vi "Update.vi"(9 "log line":string, 10 "file ref":refnum<file>, 11 "size trigger in":refnum<class "RolloverTrigger.Size.lvclass">) -> (3 "size trigger out":refnum<class "RolloverTrigger.Size.lvclass">)   [LabVIEW 2018, in "GLog.lvlib" / "RolloverTrigger.Size.lvclass"]
doc: "Updates the current file size without touching the filesystem."
uses:
  RolloverTrigger.Size.lvclass
  RolloverTrigger.Size.lvclass/RolloverTrigger.Size.ctl
panel:
  # "Connector Pane"
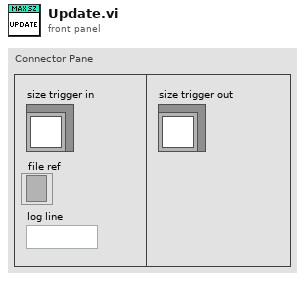
[diagram p1: front panel]
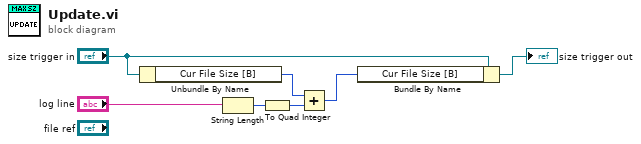
[diagram p0: block diagram]
diagram:
  n1 = Unbundle By Name("size trigger in") -> ("Cur File Size [B]"=w4:i64)
  n2 = String Length(string="log line") -> (length=w3:i32)
  n3 = To Quad Integer(1:w3) -> (0:w6:i64)
  n4 = Add(x=w4, y=w6) -> (x+y=w1:i64)
  n5 = Bundle By Name(cluster="size trigger in", "Cur File Size [B]"=w1) -> (→"size trigger out":refnum<class "RolloverTrigger.Size.lvclass">)
